vi "SPD.Common HW Setup.vi"(8 "error in (no error)":errorcluster, 10 "common hw setup":T1, 11 "SPD.Stand Ctrl in in":T2 {"spdDeviceSession"."hidSPD.Sturtup Values"."HV_bias" format="%#_6p, V"; "spdDeviceSession"."hidSPD.Sturtup Values"."TSet" format="%#_6p, DegC"; "spdDeviceSession"."hidSPD.Controller"."HV_bias" format="%#_6p, V"; "spdDeviceSession"."hidSPD.Controller"."TSet" format="%#_6p, DegC"}) -> (0 "error out":errorcluster, 3 "SPD.Stand Ctrl out":T2 {"spdDeviceSession"."hidSPD.Sturtup Values"."HV_bias" format="%#_6p, V"; "spdDeviceSession"."hidSPD.Sturtup Values"."TSet" format="%#_6p, DegC"; "spdDeviceSession"."hidSPD.Controller"."HV_bias" format="%#_6p, V"; "spdDeviceSession"."hidSPD.Controller"."TSet" format="%#_6p, DegC"})   [LabVIEW 2018]
uses:
  typedefs/SPD.Stand Ctrl.ctl
  Instruments/SPD HID Interface/hidSPDLibForLabView/LibVIs/hidSPD Controls/hidSPD Device Session.ctl
  Instruments/SPD HID Interface/hidSPDLibForLabView/LibVIs/hidSPD Controls/hidSPD.SPD specification.ctl
  Instruments/SPD HID Interface/hidSPDLibForLabView/LibVIs/hidSPD Controls/hidSPD SPD Diod Case.ctl
  Instruments/SPD HID Interface/hidSPDLibForLabView/LibVIs/hidSPD Controls/hidSPD SPD Type.ctl
  Instruments/SPD HID Interface/hidSPDLibForLabView/LibVIs/hidSPD Controls/hidSPD.STB Frequency.ctl
  Instruments/SPD HID Interface/hidSPDLibForLabView/LibVIs/hidSPD Controls/hidSPD Controller.ctl
  Instruments/KC705 DevBoard/typedefs/DevB.Session.ctl
  Instruments/KeySight 53230A/typedefs/FreqC.Session.ctl
  Instruments/KeySight 8164B/KeySight 8164B LAN InstrLib/typedefs/KeySight 8164B control.ctl
  Instruments/LeCroy SDA830/typedefs/LeCroy.Session.ctl
  typedefs/SPD.Events.ctl
  ConfigFile/SPD.Config File ctrl.ctl
  <vilib>/Utility/config.llb/Config Data RefNum.ctl
  typedefs/SPD.Meas Grid.ctl
  typedefs/SPD.Queues.ctl
  typedefs/SPD.Stand state.ctl
  typedefs/SPD.Common HW Setup ctr.ctl
  Instruments/KeySight 8164B/KeySight 8164B LAN InstrLib.lvlib
  <vilib>/Utility/config.llb/NI_LVConfig.lvlib
  Instruments/SPD HID Interface/hidSPDLibForLabView/hidSPDLibForLabView.lvlib
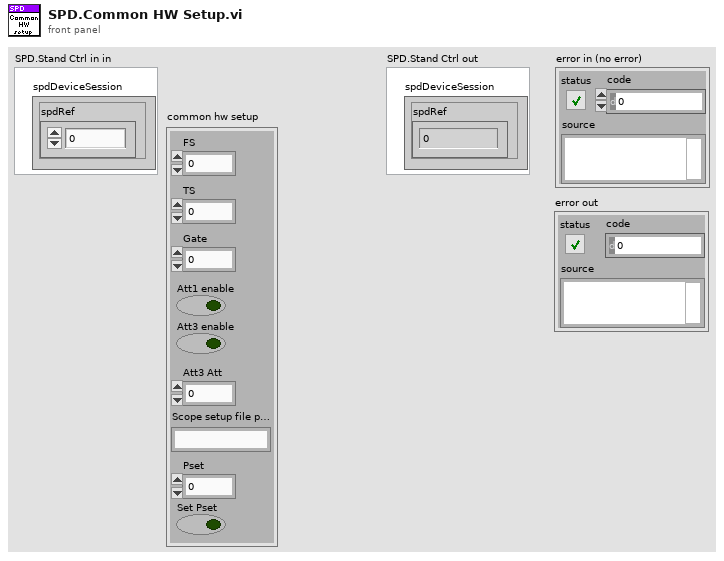
[diagram p1: front panel]
types:
  T1 = typedef "SPD.Common HW Setup ctr.ctl" = cluster{"FS":i32, "TS":i32, "Gate":dbl, "Att1 enable":bool, "Att3 enable":bool, "Att3 Att":dbl, "Scope setup file path":string, "Pset":dbl, "Set Pset":bool}
  T2 = typedef "SPD.Stand Ctrl.ctl" = cluster{"spdDeviceSession":T3, "DevBSession":T9, "FreqCSession":T10, "8164BSession":T11, "LeCroySession":T12, "Events":T13, "configFile":T14, "SPD.Meas Grid":T16, "SPD.Queues":T17, "Console":refnum<vi>}
  T3 = typedef "hidSPDLibForLabView.lvlib/hidSPD Device Session.ctl" = cluster{"spdRef":u64, "connected":bool, "spdName":string, "specification":T4, "hidSPD.Controller":T8, "hidSPD.Sturtup Values":T8}
  T4 = typedef "hidSPDLibForLabView.lvlib/hidSPD.SPD specification.ctl" = cluster{"diod case":T5, "type":T6, "frequency":T7}
  T5 = typedef "hidSPDLibForLabView.lvlib/hidSPD SPD Diod Case.ctl" = enum16{"Unknown", "default", "butterfly"}
  T6 = typedef "hidSPDLibForLabView.lvlib/hidSPD SPD Type.ctl" = enum16{"Unknown", "Free Run", "Gate"}
  T7 = typedef "hidSPDLibForLabView.lvlib/hidSPD.STB Frequency.ctl" = enum16{"Unknown", "312", "1250"}
  T8 = typedef "hidSPDLibForLabView.lvlib/hidSPD Controller.ctl" = cluster{"TSet":sgl, "HV_bias":sgl, "DDS_stb_code":u16}
  T9 = typedef "DevB.Session.ctl" = cluster{"DevBRef":refnum<visa-resource-name>, "connected":bool}
  T10 = typedef "FreqC.Session.ctl" = cluster{"FreqCRef":refnum<visa-resource-name>, "timeout":dbl, "Gate":dbl, "connected":bool}
  T11 = typedef "KeySight 8164B LAN InstrLib.lvlib/KeySight 8164B control.ctl" = cluster{"Connection ID":refnum<k5>, "Connected":bool, "Info":string, "Slots Info":string[]}
  T12 = typedef "LeCroy.Session.ctl" = cluster{"LeCroySession":refnum<visa-resource-name>, "connected":bool}
  T13 = typedef "SPD.Events.ctl" = cluster{"DCRTest":refnum<user-event>, "Stop":refnum<user-event>}
  T14 = typedef "SPD.Config File ctrl.ctl" = cluster{"configFile ref":T15, "configFile path":path, "equipmentFile ref":T15}
  T15 = typedef "NI_LVConfig.lvlib/Config Data RefNum.ctl" = refnum<k1>
  T16 = typedef "SPD.Meas Grid.ctl" = cluster{"DateTime":string, "DT":dbl[], "Insensitivity":dbl[], "Temprature":dbl[], "Stb_code":dbl[], "HV_Bias":dbl[][][][]}
  T17 = typedef "SPD.Queues.ctl" = cluster{"state queue":refnum<queue>}
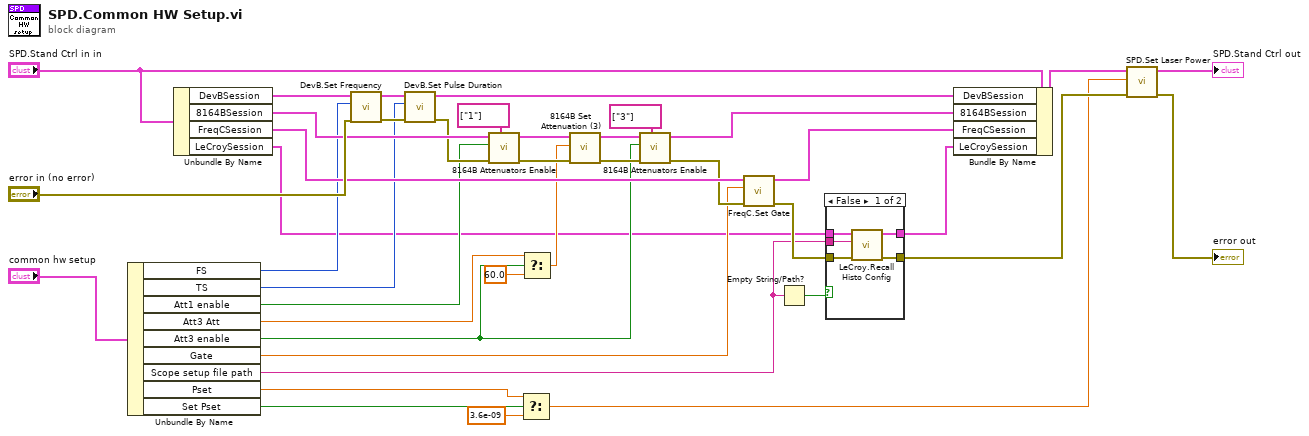
[diagram p0: block diagram]
diagram:
  n1 = Unbundle By Name("common hw setup") -> ("FS"=w25:i32, "TS"=w24:i32, "Att1 enable"=w22:bool, "Att3 Att"=w17:dbl, "Att3 enable"=w14:bool, "Gate"=w23:dbl, "Scope setup file path"=w8:string, "Pset"=w5:dbl, "Set Pset"=w6:bool)
  n2 = Unbundle By Name("SPD.Stand Ctrl in in") -> ("DevBSession"=w27:T9, "8164BSession"=w34:T11, "FreqCSession"=w35:T10, "LeCroySession"=w11:T12)
  n3 = call "DevB.Set Frequency.vi"("error in (no error)"="error in (no error)", "Frequency"=w25, "DevB Session in"=w27) -> ("error out"=w29:errorcluster, "DevB Session out"=w28:T9)  [unwired: 7 in]
  n4 = call "DevB.Set Pulse Duration.vi"("error in (no error)"=w29, "Pulse Duration"=w24, "DevB Session in"=w28) -> ("error out"=w32:errorcluster, "DevB Session out"=w36:T9)  [unwired: 7 in]
  n5 = call "8164B Attenuators Enable.vi"("Slots"=string[] ["1"], "error in"=w32, "Enable"=w22, "KeySight 8164B control in"=w34) -> ("error out"=w20:errorcluster, "KeySight 8164B control out"=w21:T11)  [unwired: 6 in]
  n6 = Select(t=w5, s=w6, f=3.6e-09) -> (s? t:f=w4:dbl)
  n7 = Select(t=w17, s=w14, f=60.0) -> (s? t:f=w16:dbl)
  n8 = call "8164B Set Attenuation (3).vi"("error in"=w20, "Att 3, dB"=w16, "KeySight 8164B control in"=w21) -> ("error out"=w19:errorcluster, "KeySight 8164B control out"=w18:T11)  [unwired: 7 in]
  n9 = call "8164B Attenuators Enable.vi"("Slots"=string[] ["3"], "error in"=w19, "Enable"=w14, "KeySight 8164B control in"=w18) -> ("error out"=w33:errorcluster, "KeySight 8164B control out"=w37:T11)  [unwired: 6 in]
  n10 = call "FreqC.Set Gate.vi"("error In"=w33, "Gate, sec"=w23, "FreqC Session in"=w35) -> ("error out"=w12:errorcluster, "FreqC Session out"=w38:T10)  [unwired: 7 in]
  n11 = Empty String/Path?(string/path=w8) -> (empty?=w9:bool)
  n12 = case shown="False" w9 {
    tunnel: w12 -> [w45 w46]
    tunnel: w11 -> [w44 w47]
    tunnel: [w43 w47] -> w10
    tunnel: [w42 w46] -> w7
    tunnel: w8 -> [w41 _]
    frame False {
      n13 = call "LeCroy.Recall Histo Config.vi"("Error In"=w45, "Filename (panel.lss)"=w41, "LeCroy.Session in"=w44) -> ("Error Out"=w42:errorcluster, "LeCroy.Session out"=w43:T12)  [unwired: 7 in]
    }
    frame True {
    }
  }
  n14 = Bundle By Name(cluster="SPD.Stand Ctrl in in", "DevBSession"=w36, "8164BSession"=w37, "FreqCSession"=w38, "LeCroySession"=w10) -> (w13:T2)
  n15 = call "SPD.Set Laser Power.vi"("Error In"=w7, "Pset"=w4, "SPD.Stand Ctrl in"=w13) -> ("Error Out"=→"error out":errorcluster, "SPD.Stand Ctrl out"=→"SPD.Stand Ctrl out":T2)  [unwired: 7 in]
